vi "parseSettingsLine.vi"(11 "String":string) -> (1 "comment":string, 2 "value":string, 3 "key":string)   [LabVIEW 2019, in "Controller.lvclass"]
uses:
  Controller.lvclass
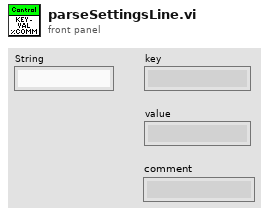
[diagram p1: front panel]
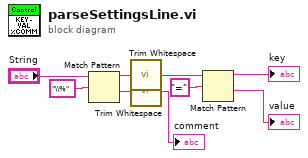
[diagram p0: block diagram]
diagram:
  n1 = Match Pattern(string="String", regular expression="\\%") -> (before substring=w7:string, after substring=w2:string)  [unwired: 1 in, 2 out]
  n2 = call <vilib>:"Trim Whitespace.vi"("string"=w7) -> ("trimmed string"=w9:string)  [unwired: 1 in]
  n3 = call <vilib>:"Trim Whitespace.vi"("string"=w2) -> ("trimmed string"=→"comment":string)  [unwired: 1 in]
  n4 = Match Pattern(string=w9, regular expression="=") -> (before substring=→"key":string, after substring=→"value":string)  [unwired: 1 in, 2 out]
